vi "m10.wfg.vi"(0 "Stimulus Type":u16(ring) items=["Off", "DC", "Noise", "PT", "FM"], 1 "Param 0":dbl, 2 "Param 1":dbl, 3 "Param 2":dbl, 4 "Param 3":dbl, 5 "error in (no error)":errorcluster, 8 "Waveform Properties":T1 {"Ramp (s)" min=0.0; "Fs (Hz)" min=0.0}) -> (14 "Waveform Out":waveform(dbl), 19 "error out":errorcluster)   [LabVIEW 2009]
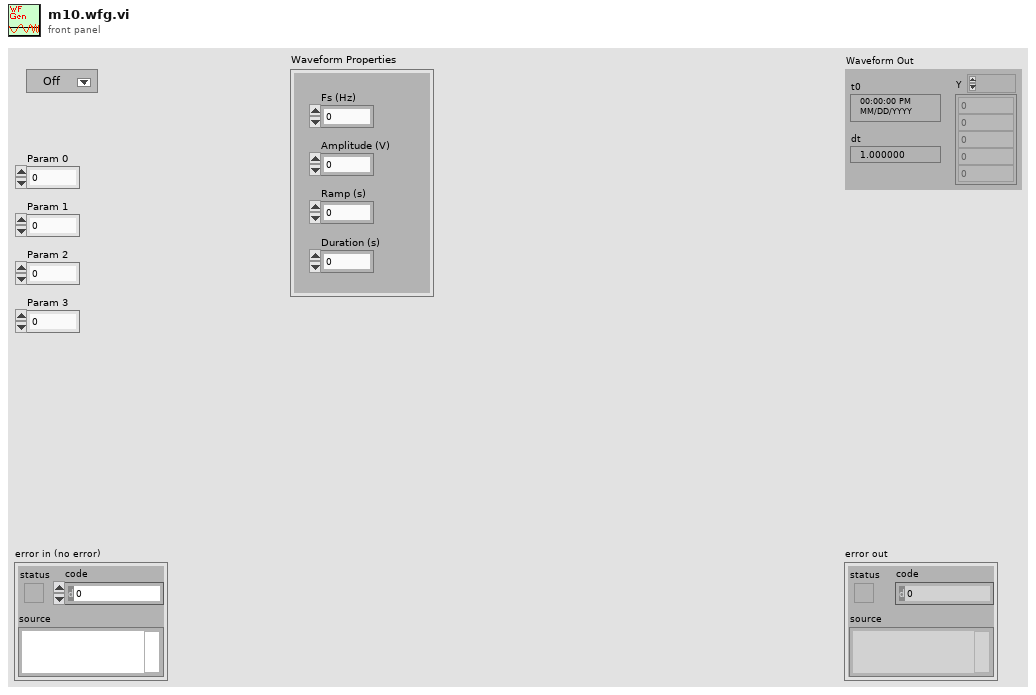
[diagram p1: front panel]
types:
  T1 = cluster{"Fs (Hz)":dbl, "Amplitude (V)":dbl, "Ramp (s)":dbl, "Duration (s)":dbl}
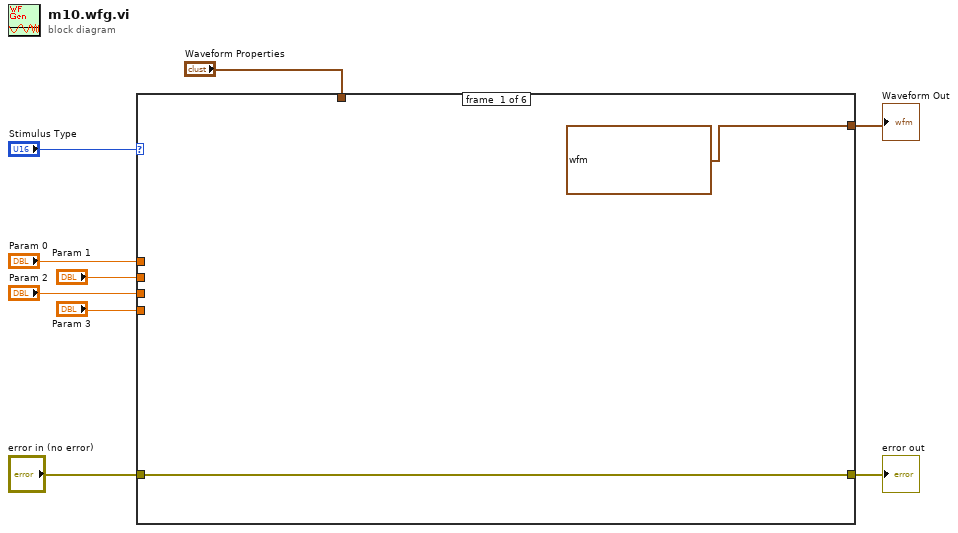
[diagram p0: block diagram]
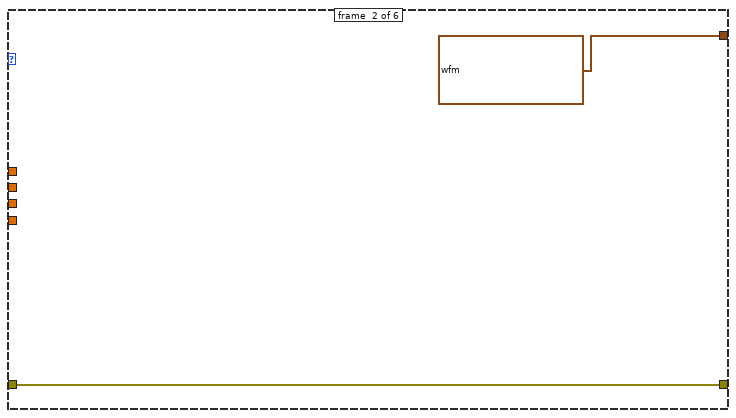
[diagram p2: hidden frame]
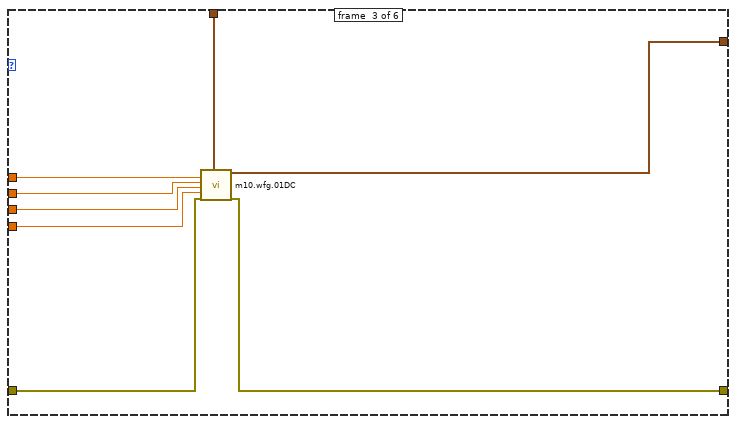
[diagram p3: hidden frame]
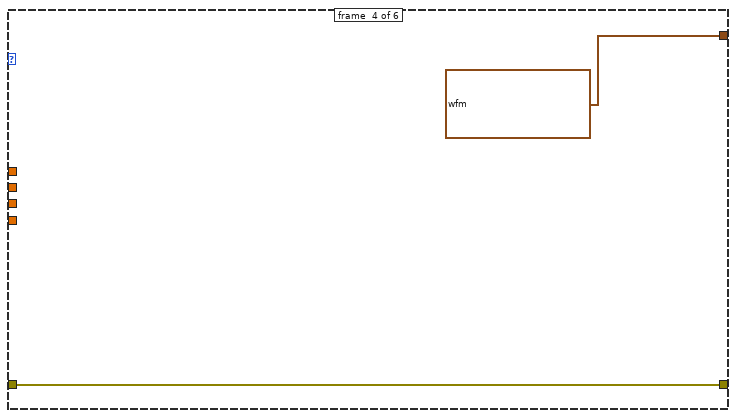
[diagram p4: hidden frame]
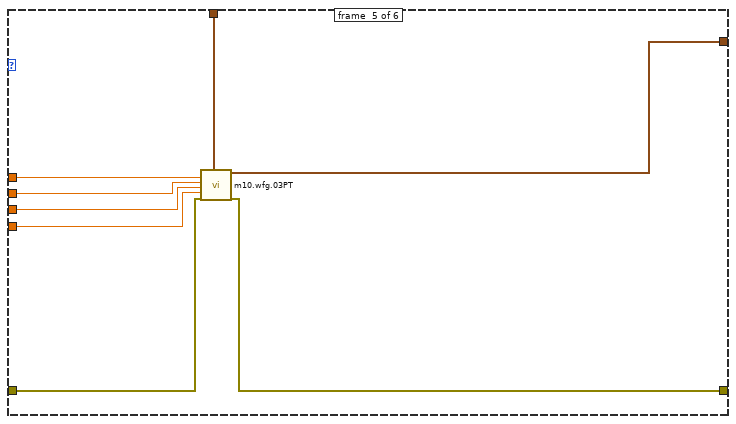
[diagram p5: hidden frame]
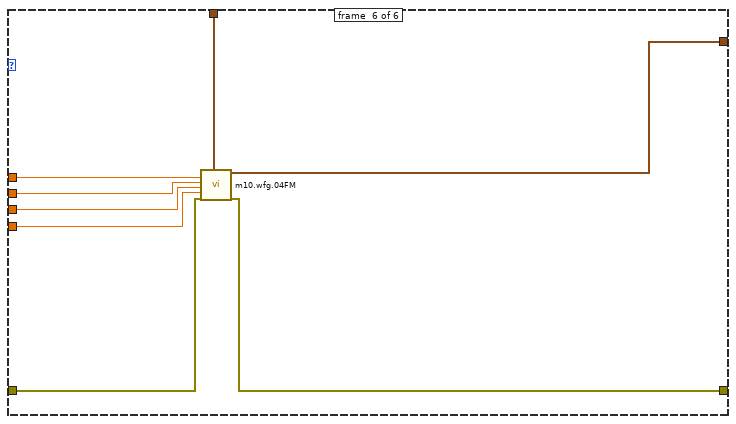
[diagram p6: hidden frame]
diagram:
  n1 = case shown="1000, Default" "Stimulus Type" {
    tunnel: "Param 0" -> [_ _ w21 _ w31 w39]
    tunnel: "Param 1" -> [_ _ w20 _ w30 w38]
    tunnel: "Param 2" -> [_ _ w19 _ w29 w37]
    tunnel: "Param 3" -> [_ _ w18 _ w28 w36]
    tunnel: "Waveform Properties" -> [_ _ w14 _ w24 w32]
    tunnel: "error in (no error)" -> [w10 w12 w17 w23 w27 w35]
    tunnel: [w10 w12 w16 w23 w26 w34] -> w2
    tunnel: [waveform(dbl) ? ("Waveform") waveform(dbl) ? ("Waveform") w15 waveform(dbl) ? ("Waveform") w25 w33] -> w1
    frame #0 {
    }
    frame #1 {
    }
    frame #2 {
      n2 = call "m10.wfg.01DC.vi"("Param 0"=w21, "Param 1"=w20, "Param 2"=w19, "Param 3"=w18, "error in (no error)"=w17, "Waveform Properties"=w14) -> ("Waveform Out"=w15:waveform(dbl), "error out"=w16:errorcluster)  [unwired: 12 in]
    }
    frame #3 {
    }
    frame #4 {
      n3 = call "m10.wfg.03PT.vi"("Param 0"=w31, "Param 1"=w30, "Param 2"=w29, "Param 3"=w28, "error in (no error)"=w27, "Waveform Properties"=w24) -> ("Waveform Out"=w25:waveform(dbl), "error out"=w26:errorcluster)  [unwired: 12 in]
    }
    frame #5 {
      n4 = call "m10.wfg.04FM.vi"("Param 0"=w39, "Param 1"=w38, "Param 2"=w37, "Param 3"=w36, "error in (no error)"=w35, "Waveform Properties"=w32) -> ("Waveform Out"=w33:waveform(dbl), "error out"=w34:errorcluster)  [unwired: 12 in]
    }
  }
  "Waveform Out" <- w1
  "error out" <- w2
